vi "sub_strain-cal.vi"(11 "wf in":waveform(dbl)[](array[waveform])) -> (3 "wf out":waveform(dbl)[](array[waveform]))   [LabVIEW 2013]
panel:
  in  "Interpolation Points":dbl[][](array[numeric]) caption="보간 포인트" format="%#.6f"
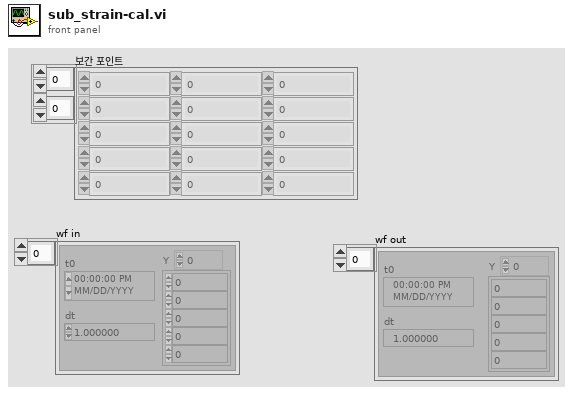
[diagram p1: front panel]
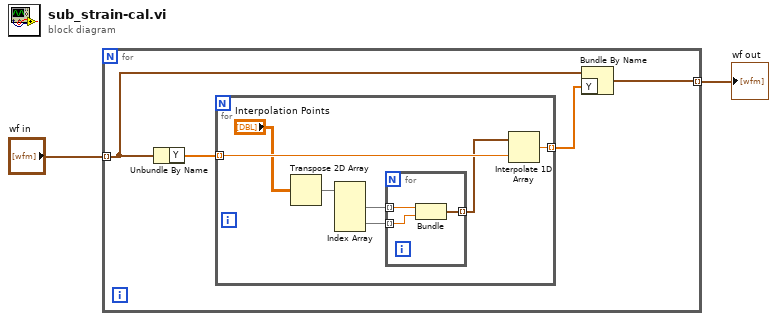
[diagram p0: block diagram]
diagram:
  n1 = for {
    tunnel: [w3] -> w2 mode=indexing
    tunnel: "wf in" -> [w6] mode=indexing
    n2 = Unbundle By Name(w6) -> ("Y"=w4:dbl[])
    n3 = for {
      tunnel: [w13] -> w5 mode=indexing
      tunnel: w4 -> [w12] mode=indexing
      n4 = Transpose 2D Array(2D array="Interpolation Points") -> (transposed array=w9:dbl[][])
      n5 = Index Array(array=w9) -> (element #1=w11:dbl[], element #2=w10:dbl[])  [unwired: 4 in]
      n6 = for {
        tunnel: w11 -> [w16] mode=indexing
        tunnel: w10 -> [w15] mode=indexing
        tunnel: [w14] -> w7 mode=indexing
        n7 = Bundle(w16, w15) -> (w14:cluster{dbl, dbl})  [unwired: 1 in]
      }
      n8 = Interpolate 1D Array(1:w12, 2:w7) -> (0:w13:dbl)
    }
    n9 = Bundle By Name(cluster=w6, "Y"=w5) -> (w3:waveform(dbl))
  }
  "wf out" <- w2
